vi "data-center-simulator-events.vi"() -> ()   [LabVIEW 2024]
uses:
  <resource>/objmgr/daqmx.rc
  <vilib>/DAQmx/create/channels.llb/DAQmx Create Channel (AO-Voltage-Basic).vi
  <vilib>/DAQmx/configure/timing.llb/DAQmx Timing (Sample Clock).vi
  <vilib>/DAQmx/write.llb/DAQmx Write (Analog 1D Wfm NChan NSamp).vi
panel:
  in  "Quit":bool
  in  "Start":bool
  in  "Stop":bool
  in  "Tab Control":T1(tab)=enum."Power Signals"
  in  "Generation Type":T2(ring)=enum."Voltage Only (3V)"
  in  "Maximum Value":dbl=10.0 format="%0.2f"
  in  "Minimum Value":dbl=-10.0 format="%0.2f"
  in  "Physical Channels":tag="cDAQ1Mod1/ao0:2"
  in  "Sample Clock Rate":dbl=20000.0 format="%0.2f"
  out "Actual Sample Clock Rate":dbl format="%.2f"
  in  "Harmonics":T3(array[cluster])
  in  "Fundamental":cluster{"level (%)":dbl, "phase (°)":dbl}[](array[cluster])=[{"level (%)"=100.0, "phase (°)"=0.0}, {"level (%)"=100.0, "phase (°)"=240.0}, {"level (%)"=100.0, "phase (°)"=120.0}, {"level (%)"=100.0, "phase (°)"=0.0}, {"level (%)"=100.0, "phase (°)"=240.0}, {"level (%)"=100.0, "phase (°)"=120.0}, {"level (%)"=1.0, "phase (°)"=35.0}]
  in  "Frequency and Amplitude":T4={"frequency (Hz)"=60.0, "voltage (V) RMS"=1.50975, "current (A) RMS"=0.1875} {"current (A) RMS" scale=0.0..5.0; "voltage (V) RMS" scale=0.0..5.0; "frequency (Hz)" scale=55.0..65.0}
  in  "Generate Event":bool
  in  "Level (%)":dbl
  in  "Signal":enum16{"Voltage A", "Voltage B", "Voltage C"}(ring)
  out "System Waveform Graph 2":waveform(dbl)(graph)={"t0"=timestamp(0 s since 1904-01-01), "dt"=5e-05, "Y"=array[5000 elements]} caption="Event Waveform"
  out "System Waveform Graph":waveform(dbl)[](graph)=[{"t0"=timestamp(0 s since 1904-01-01), "dt"=5e-05, "Y"=array[5000 elements]}, {"t0"=timestamp(0 s since 1904-01-01), "dt"=5e-05, "Y"=array[5000 elements]}] caption="Output Waveform"
  # "Va"
  # "Vb"
  # "Vc"
  # "Ia"
  # "Ib"
  # "Ic"
  # "In"
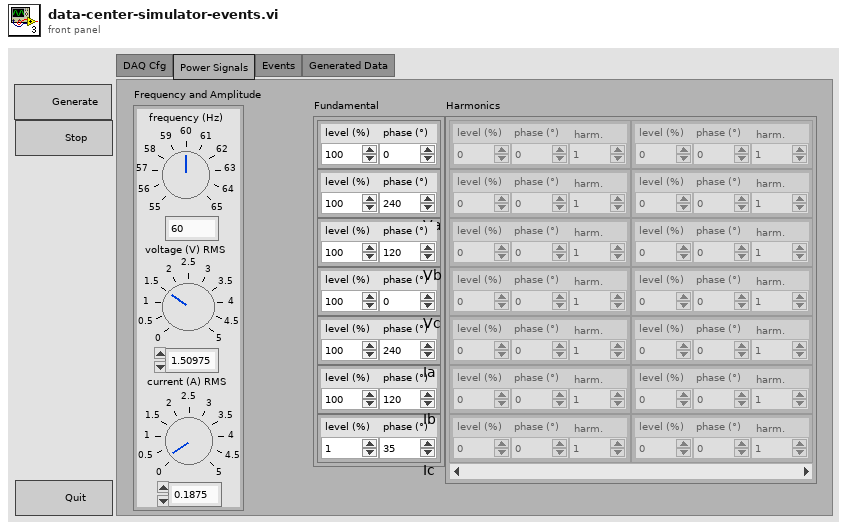
[diagram p1: front panel]
types:
  T1 = enum32{"DAQ Cfg", "Power Signals", "Events", "Generated Data"}
  T2 = enum16{"Single Phase (1V + 1I)", "Voltage Only (3V)", "Three Phase (3V + 4I)"}
  T3 = cluster{"level (%)":dbl, "phase (°)":dbl, "harm.":dbl}[][]
  T4 = cluster{"frequency (Hz)":sgl, "voltage (V) RMS":dbl, "current (A) RMS":dbl}
  T5 = typedef "AMC.lvlib/Message Queue.ctl" = refnum<queue>
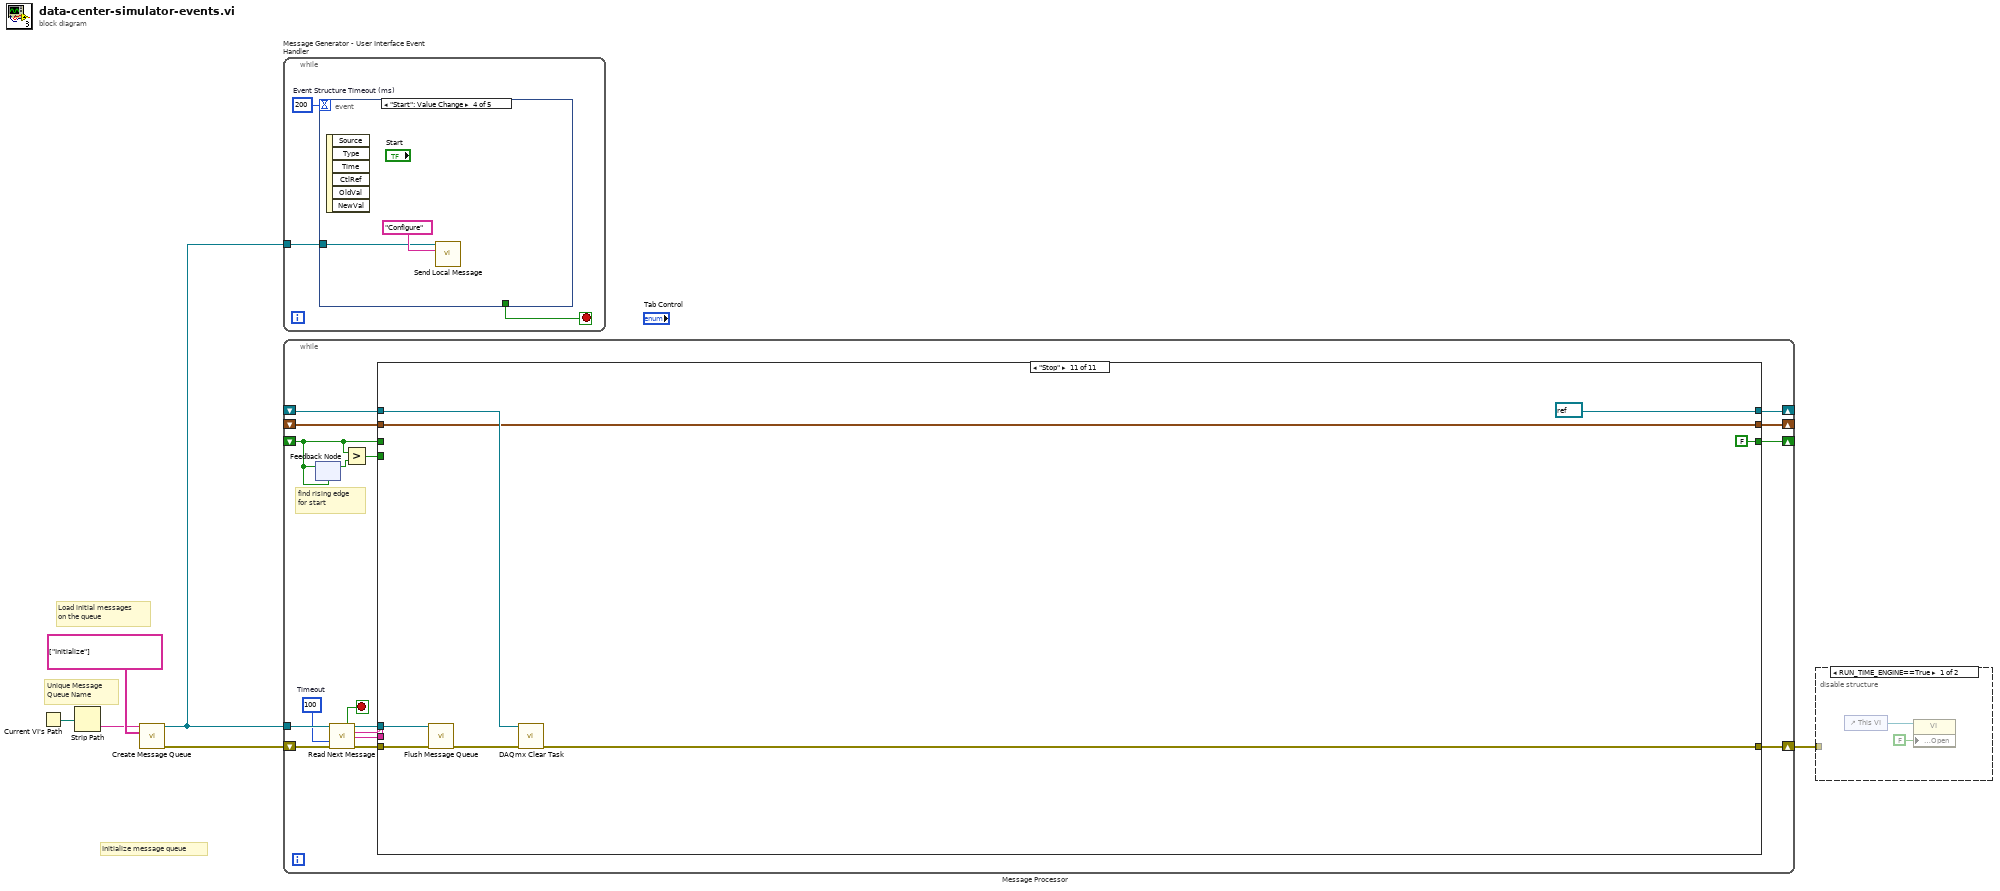
[diagram p0: block diagram]
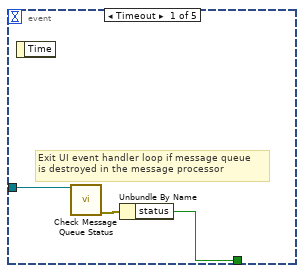
[diagram p3: hidden frame]
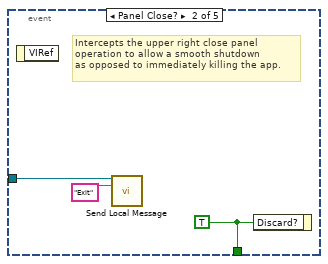
[diagram p4: hidden frame]
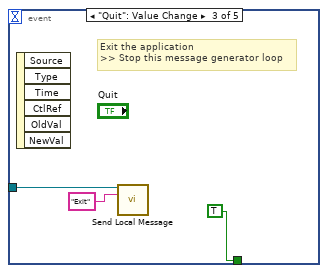
[diagram p5: hidden frame]
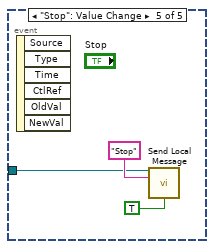
[diagram p6: hidden frame]
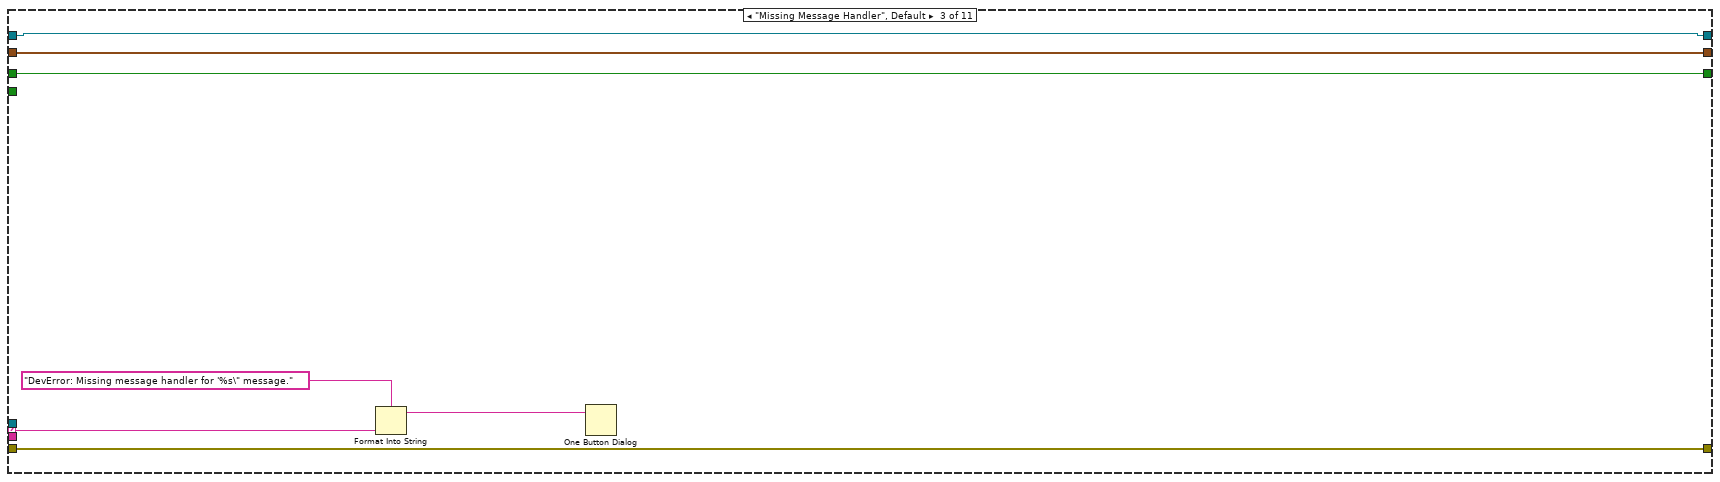
[diagram p9: hidden frame]
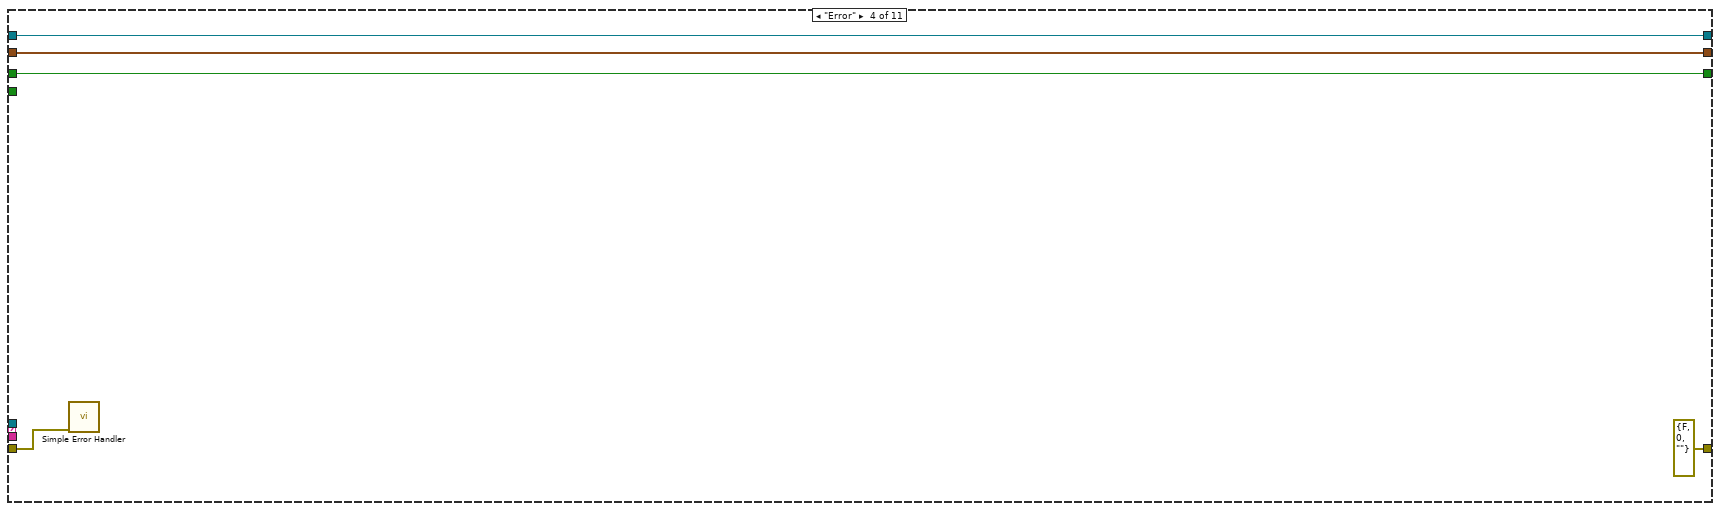
[diagram p10: hidden frame]
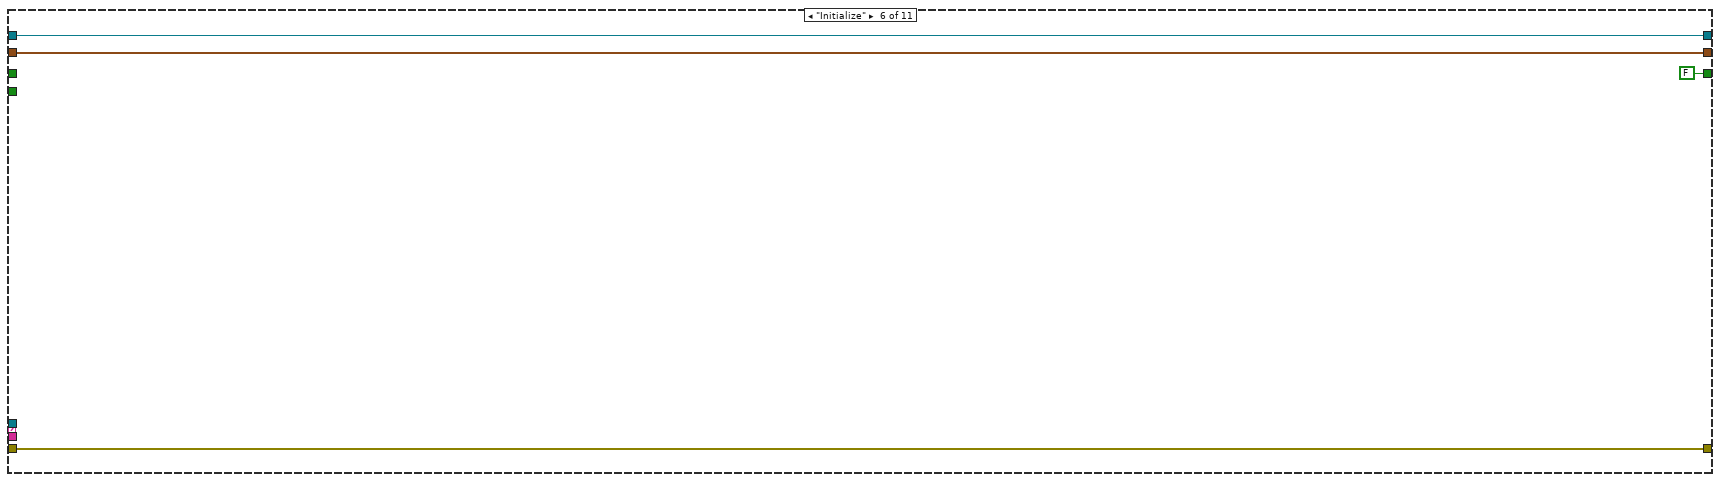
[diagram p12: hidden frame]
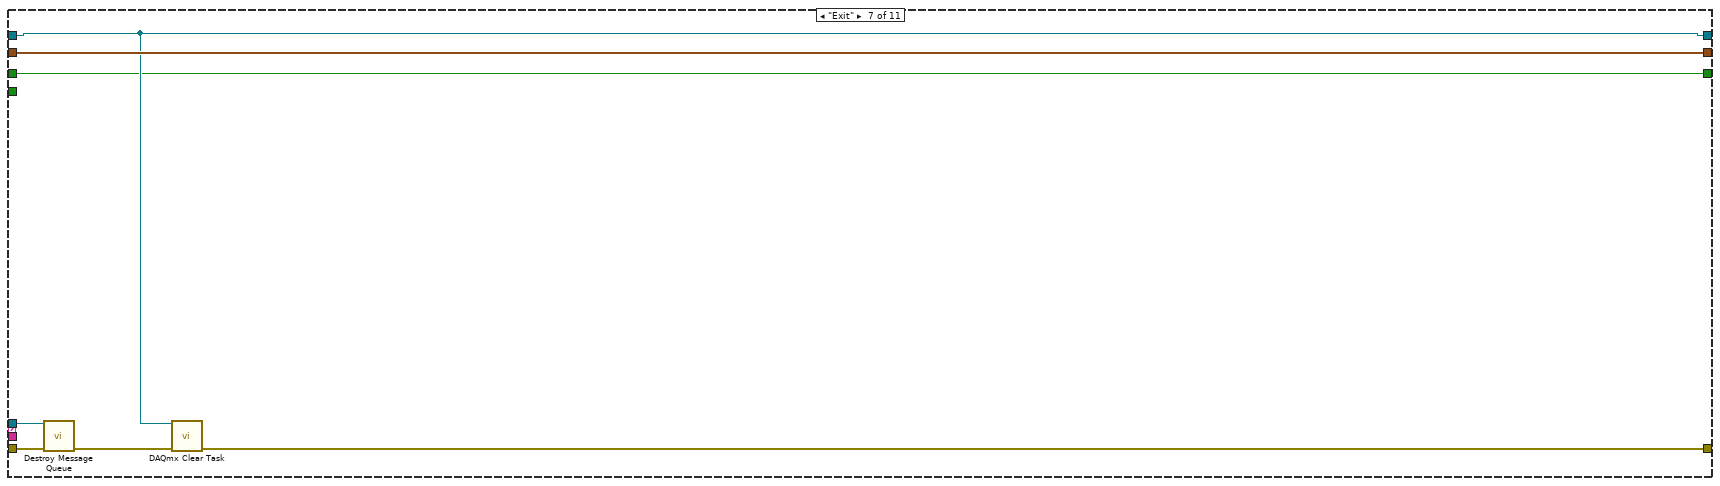
[diagram p13: hidden frame]
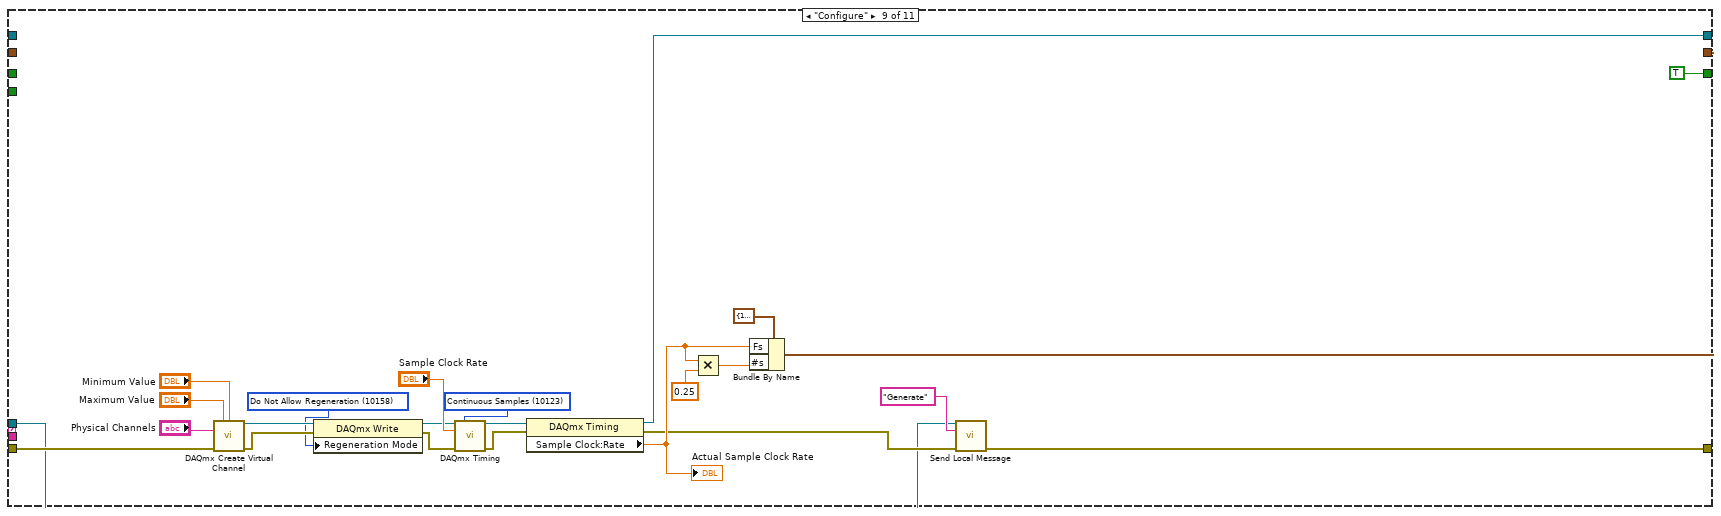
[diagram p15: hidden frame]
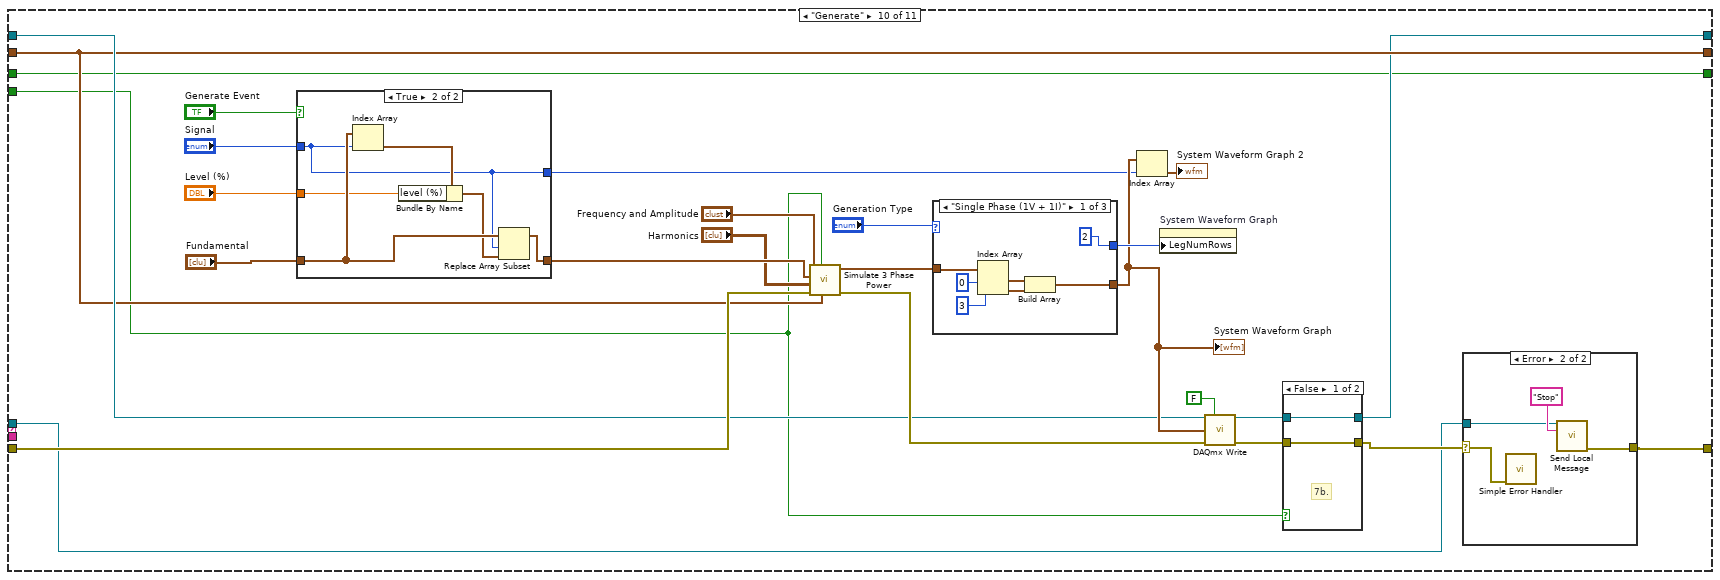
[diagram p16: hidden frame]
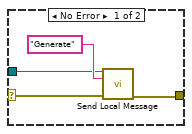
[diagram p17: hidden frame]
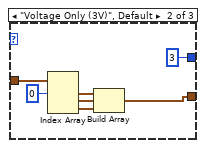
[diagram p18: hidden frame]
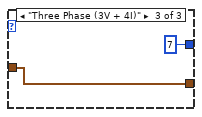
[diagram p19: hidden frame]
diagram:
  # "Initialize message queue"
  # "Unique Message\nQueue Name"
  # "Load initial messages\non the queue"
  n1 = Current VI's Path() -> (path=w2:path)
  n2 = Strip Path(path=w2) -> (name=w5:string)  [unwired: 1 out]
  n3 = call <vilib>:"Create Message Queue.vi"("message queue name"=w5, "initial message names"=string[] ["Initialize"]) -> ("message queue out"=w4:T5, "error out"=w3:errorcluster)  [unwired: 12 in]
  n4 = while "Message Generator - User Interface Event Handler" {
    tunnel: w4 -> [w7]
    stop <- w8 stop-if-true
    w9 = 200  # Event Structure Timeout (ms)
    n5 = event shown="[3] \"Start\": Value Change" {
      selector: _ -> [_ _ _ _ _]
      dyn-events: _ -> [_ _ _ _ _]
      timeout: w9 -> [_ _ _ _ _]
      tunnel: [w10 w15 TRUE ("Discard?") _ _] -> w8
      tunnel: w7 -> [w11 w13 w16 w19 w21]
      event Timeout {
        # "Exit UI event handler loop if message queue\nis destroyed in the message processor"
        n6 = event-data() -> ()  [unwired: 2 out]
        n7 = call <vilib>:"Check Message Queue Status.vi"("message queue in"=w11) -> ("error out"=w12:errorcluster)  [unwired: 10 in, 4 out]
        n8 = Unbundle By Name(w12) -> ("status"=w10:bool)
      }
      event Panel Close? {
        w15 = TRUE ("Discard?")
        # "Intercepts the upper right close panel\noperation to allow a smooth shutdown\nas opposed to immediately killing the app."
        n9 = event-data() -> ()  [unwired: 2 out]
        n10 = call <vilib>:"Send Local Message.vi"("message queue in"=w13, "message name"="Exit") -> ()  [unwired: 11 in, 3 out]
        n11 = event-data("Discard?"=w15) -> ()  [unwired: 1 in, 1 out]
      }
      event "Quit": Value Change {
        # "Exit the application\n>> Stop this message generator loop"
        n12 = event-data() -> ()  [unwired: 7 out]
        n13 = call <vilib>:"Send Local Message.vi"("message queue in"=w16, "message name"="Exit") -> ()  [unwired: 11 in, 3 out]
      }
      event "Start": Value Change {
        n14 = event-data() -> ()  [unwired: 7 out]
        n15 = call <vilib>:"Send Local Message.vi"("message queue in"=w19, "message name"="Configure") -> ()  [unwired: 11 in, 3 out]
      }
      event "Stop": Value Change {
        n16 = event-data() -> ()  [unwired: 7 out]
        n17 = call <vilib>:"Send Local Message.vi"("message queue in"=w21, "message name"="Stop", "priority message (F)"=TRUE ("Priority Message (F)")) -> ()  [unwired: 10 in, 3 out]
      }
    }
  }
  n18 = while "Message Processor" {
    shift-left: w3 -> [w36]
    shift-right: [w40] -> w1
    tunnel: w4 -> [w37]
    shift-right: [w31] -> _
    shift-left: _ -> [w30]
    shift-right: [w29] -> _
    shift-left: _ -> [w28]
    shift-right: [w27] -> _
    shift-left: _ -> [w24]
    stop <- w39 stop-if-true
    w32 = 100  # Timeout
    # "find rising edge\nfor start"
    n19 = feedback #1(w24) -> (w26:bool)
    n20 = feedback-in #1(w24) -> ()
    n21 = call <vilib>:"Read Next Message.vi"("message queue in"=w37, "timeout (1 ms)"=w32, "error in"=w36) -> ("exit process?"=w39:bool, "message queue out"=w38:T5, "message name"=w34:string, "message value"=w33:string, "error out"=w35:errorcluster)  [unwired: 5 in, 3 out]
    n22 = Greater?(x=w24, y=w26) -> (0:w25:bool)
    n23 = case shown="\"Stop\"" w34 {
      selector: w34 -> [_ _ w54 _ _ _ _ _ _ _ _]
      tunnel: w38 -> [_ _ _ _ _ _ w74 _ w82 w106 w172]
      tunnel: w35 -> [w44 w48 w55 w60 w64 w68 w75 w79 w87 w112 w173]
      tunnel: [w44 w48 w55 errorcluster {"status"=FALSE, "code"=0, "source"=""} ("error out") w64 w68 w71 w79 w81 w107 w168] -> w40
      tunnel: w33 -> [_ _ _ _ _ _ _ _ _ _ _]
      tunnel: [w42 w46 w50 w58 w62 w66 w70 w77 w86 w109 refnum<k21> refnum ("task out")] -> w31
      tunnel: w30 -> [w42 w46 w50 w58 w62 w66 w70 w77 _ w111 w171]
      tunnel: [w43 w47 w51 w59 w63 w67 w73 w78 w85 w110 w169] -> w29
      tunnel: w28 -> [w43 w47 w51 w59 w63 w67 w73 w78 _ w110 w169]
      tunnel: [w41 w45 w49 w56 w61 FALSE w69 w76 TRUE w104 FALSE] -> w27
      tunnel: w24 -> [w41 w45 w49 w56 w61 _ w69 w76 _ w104 _]
      tunnel: w25 -> [_ _ _ _ _ _ _ _ _ w105 _]
      frame "---------- Framework Operations ----------" {
      }
      frame "", "Idle" {
      }
      frame "Missing Message Handler", Default {
        n24 = Format Into String(format string="DevError: Missing message handler for '%s\" message." ("message"), w54) -> (resulting string=w52:string)  [unwired: 2 in, 1 out]
        n25 = One Button Dialog(message=w52) -> ()  [unwired: 2 out]
      }
      frame "Error" {
        n26 = call <vilib>:"Simple Error Handler.vi"("error in (no error)"=w60) -> ()  [unwired: 1 in, 8 out]
      }
      frame "---------- Generic Operations ----------" {
      }
      frame "Initialize" {
      }
      frame "Exit" {
        n27 = call <vilib>:"Destroy Message Queue.vi"("message queue in"=w74, "error in"=w75) -> ("error out"=w72:errorcluster)  [unwired: 11 in, 2 out]
        n28 = call <vilib>:"DAQmx Clear Task.vi"("task in"=w70, "error in"=w72) -> ("error out"=w71:errorcluster)  [unwired: 13 in]
      }
      frame "---------- Application Operations ----------" {
        # "Dummy case to add a seperator in the Case Structure menu"
      }
      frame "Configure" {
        w89 = 10158 items=["Allow Regeneration"=10097, "Do Not Allow Regeneration"=10158] ("RegenMode")
        w88 = 10123 items=["Finite Samples"=10178, "Continuous Samples"=10123] ("sample mode")
        n29 = call-poly <vilib>:"DAQmx Create Virtual Channel.vi"("maximum value"="Maximum Value", "minimum value"="Minimum Value", "physical channels"="Physical Channels", "error in"=w87) -> ("task out"=w97:refnum<k21>, "error out"=w98:errorcluster)  [unwired: 10 in]
        n30 = property class="DAQmx Write"(reference=w97, error in=w98, "Regeneration Mode"=w89) -> (reference out=w99:refnum<k21>, error out=w100:errorcluster)
        n31 = call-poly <vilib>:"DAQmx Timing.vi"("task/channels in"=w99, "sample mode"=w88, "rate"="Sample Clock Rate", "error in"=w100) -> ("task out"=w95:refnum<k21>, "error out"=w96:errorcluster)  [unwired: 10 in]
        n32 = property class="DAQmx Timing"(reference=w95, error in=w96) -> (reference out=w86:refnum<k21>, error out=w83:errorcluster, "Sample Clock:Rate"=w102:dbl)
        "Actual Sample Clock Rate" <- w102
        n33 = Multiply(x=w102, y=0.25) -> (x*y=w103:dbl)
        n34 = Bundle By Name(cluster=cluster{"Fs":dbl, "#s":dbl} {"Fs"=1000.0, "#s"=1000.0} ("sampling info"), "Fs"=w102, "#s"=w103) -> (w85:cluster{"Fs":dbl, "#s":dbl})
        n35 = call <vilib>:"Send Local Message.vi"("message queue in"=w82, "message name"="Generate" ("Message Name"), "error in"=w83) -> ("error out"=w81:errorcluster)  [unwired: 10 in, 2 out]
      }
      frame "Generate" {
        n36 = case shown="True" "Generate Event" {
          tunnel: "Fundamental" -> [w154 w159]
          tunnel: "Signal" -> [_ w155]
          tunnel: [w154 w158] -> w122
          tunnel: "Level (%)" -> [_ w156]
          tunnel: [_ w155] -> w125
          frame False {
          }
          frame True {
            n37 = Index Array(array=w159, index=w155) -> (element=w160:cluster{"level (%)":dbl, "phase (°)":dbl})
            n38 = Bundle By Name(cluster=w160, "level (%)"=w156) -> (w157:cluster{"level (%)":dbl, "phase (°)":dbl})
            n39 = Replace Array Subset(array=w159, new element=w157, index=w155) -> (w158:cluster{"level (%)":dbl, "phase (°)":dbl}[])
          }
        }
        n40 = call "Simulate 3 Phase Power.vi"("sampling info"=w110, "Reset"=w105, "error in"=w112, "Harmonics Array"="Harmonics", "Fundamental Array"=w122, "Frequency and Amplitude"="Frequency and Amplitude") -> ("error out"=w115:errorcluster, "Wfm data"=w126:waveform(dbl)[])  [unwired: 4 in]
        n41 = case shown="\"Single Phase (1V + 1I)\"" "Generation Type" {
          tunnel: w126 -> [w143 w151 w153]
          tunnel: [w140 w147 w153] -> w127
          tunnel: [2 3 7] -> w129
          frame "Single Phase (1V + 1I)" {
            n42 = Index Array(array=w143, index #1=0 ("index"), index #2=3 ("index")) -> (element #1=w142:waveform(dbl), element #2=w141:waveform(dbl))
            n43 = Build Array(w142, w141) -> (w140:waveform(dbl)[])
          }
          frame "Voltage Only (3V)", Default {
            n44 = Index Array(array=w151, index #1=0 ("index")) -> (element #1=w149:waveform(dbl), element #2=w148:waveform(dbl), element #3=w146:waveform(dbl))  [unwired: 2 in]
            n45 = Build Array(w149, w148, w146) -> (w147:waveform(dbl)[])
          }
          frame "Three Phase (3V + 4I)" {
          }
        }
        "System Waveform Graph" <- w127
        n46 = Index Array(array=w127, index=w125) -> (element=→"System Waveform Graph 2":waveform(dbl))
        n47 = property on="System Waveform Graph" class="WFGraph (strict)"("LegNumRows"=w129) -> ()  [unwired: 2 in, 2 out]
        n48 = call-poly <vilib>:"DAQmx Write.vi"("task/channels in"=w111, "auto start"=FALSE, "data"=w127, "error in"=w115) -> ("task out"=w113:refnum<k21>, "error out"=w114:errorcluster)  [unwired: 9 in, 1 out]
        n49 = case shown="False" w105 {
          tunnel: w113 -> [w162 w166]
          tunnel: w114 -> [w161 w165]
          tunnel: [w161 w164] -> w108
          tunnel: [w162 w163] -> w109
          frame False {
            # "7b."
          }
          frame True {
            n50 = call <vilib>:"DAQmx Start Task.vi"("task/channels in"=w166, "error in"=w165) -> ("task out"=w163:refnum<k21>, "error out"=w164:errorcluster)  [unwired: 12 in]
          }
        }
        n51 = case shown="Error" w108 {
          selector: w108 -> [w132 w134]
          tunnel: [w130 w135] -> w107
          tunnel: w106 -> [w131 w136]
          frame No Error {
            n52 = call <vilib>:"Send Local Message.vi"("message queue in"=w131, "message name"="Generate" ("Message Name"), "error in"=w132) -> ("error out"=w130:errorcluster)  [unwired: 10 in, 2 out]
          }
          frame Error {
            n53 = call <vilib>:"Simple Error Handler.vi"("error in (no error)"=w134) -> ()  [unwired: 1 in, 8 out]
            n54 = call <vilib>:"Send Local Message.vi"("message queue in"=w136, "message name"="Stop" ("Message Name")) -> ("error out"=w135:errorcluster)  [unwired: 11 in, 2 out]
          }
        }
      }
      frame "Stop" {
        n55 = call <vilib>:"Flush Message Queue.vi"("message queue in"=w172, "error in"=w173) -> ("error out"=w174:errorcluster)  [unwired: 11 in, 2 out]
        n56 = call <vilib>:"DAQmx Clear Task.vi"("task in"=w171, "error in"=w174) -> ("error out"=w168:errorcluster)  [unwired: 13 in]
      }
    }
  }
  n57 = disable-structure shown="RUN_TIME_ENGINE==True" {
    disable-tunnel: w1 -> [_ _]
    frame condition #0 {
      n58 = control-ref of="This VI"() -> (w176:refnum<vi>)
      n59 = property class="VI"(reference=w176, "Front Panel.Open"=FALSE ("Front Panel Window:Open")) -> ()  [unwired: 1 in, 2 out]
    }
    frame condition #1 (active) {
    }
  }
